vi "JKISM++ Check If Module Exists.vi"(8 "Error in":errorcluster caption="Error in (no error)", 11 "JKISM Name":string) -> (0 "Error out":errorcluster, 2 "Exist?":bool, 3 "JKISM Name(dup)":string)   [LabVIEW 2014, in "JKI State Machine++.lvlib"]
doc: "Check if module with specified name exists.\n\n<b>Inputs:</b>\n - <b>JKISM Name</b>: JKISM Module Name\n - <b>Error in</b>: Error cluster\n\n<b>Outputs:</b>\n - <b>Exist?</b>: Return True if spcified module exists.\n - <b>JKISM Name(dup)</b>: Return <b>JKISM Name</b>\n - <b>Error out</b>: Error cluster"
uses:
  JKI State Machine++.lvlib
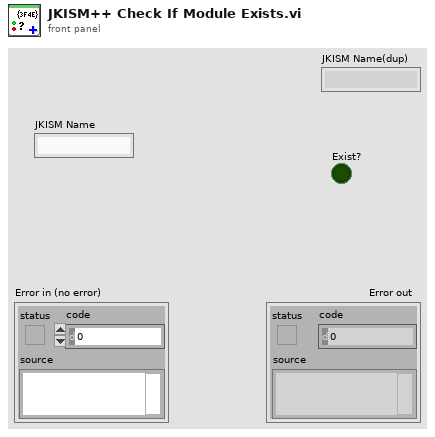
[diagram p1: front panel]
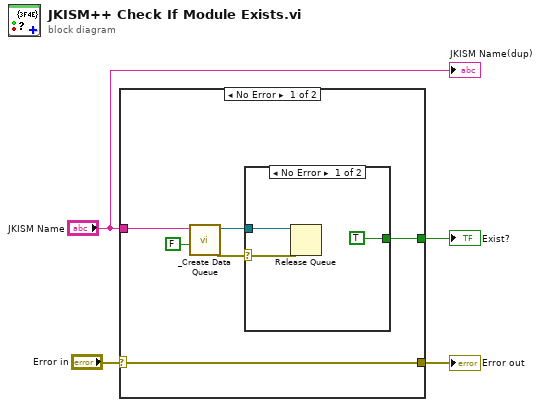
[diagram p0: block diagram]
diagram:
  n1 = case shown="No Error" "Error in" {
    selector: "Error in" -> [w5 w14]
    tunnel: "JKISM Name" -> [w10 _]
    tunnel: [w6 _] -> w3
    tunnel: [w5 w14] -> w1
    frame No Error {
      n2 = call "_Create Data Queue.vi"("create if not found? (T)"=FALSE, "Name"=w10) -> ("error out"=w8:errorcluster, "Queue out"=w7:refnum<queue>)  [unwired: 7 in, 1 out]
      n3 = case shown="No Error" w8 {
        selector: w8 -> [w12 _]
        tunnel: w7 -> [w13 _]
        tunnel: [TRUE _] -> w6
        frame No Error {
          n4 = Release Queue(queue=w13, error in (no error)=w12) -> ()  [unwired: 1 in, 3 out]
        }
        frame Error {
        }
      }
    }
    frame Error {
    }
  }
  "Error out" <- w1
  "Exist?" <- w3
  "JKISM Name(dup)" <- "JKISM Name"
